vi "Launch New Client Proxy.vi"(8 "error in (no error)":errorcluster, 9 "Client Proxy LNA":refnum<class "Client Proxy LNA.lvclass">, 10 "remote address":string, 11 "Server Controller in":refnum<class "Server Controller.lvclass">) -> (0 "error out":errorcluster, 3 "Server Controller out":refnum<class "Server Controller.lvclass">)   [LabVIEW 2016]
uses:
  Server Controller.lvclass
  Client Proxy LNA/Client Proxy LNA.lvclass
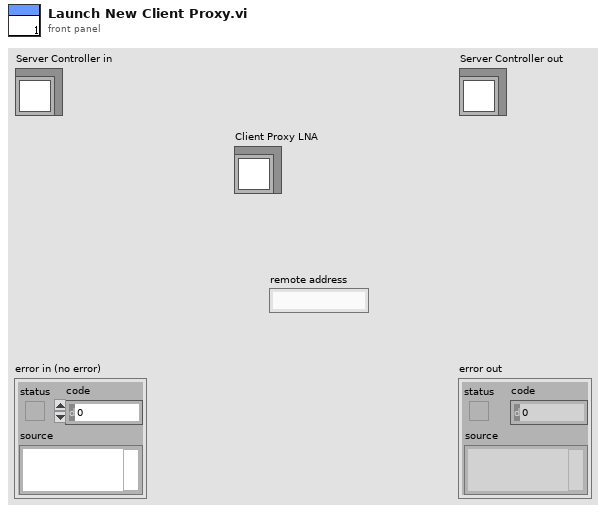
[diagram p1: front panel]
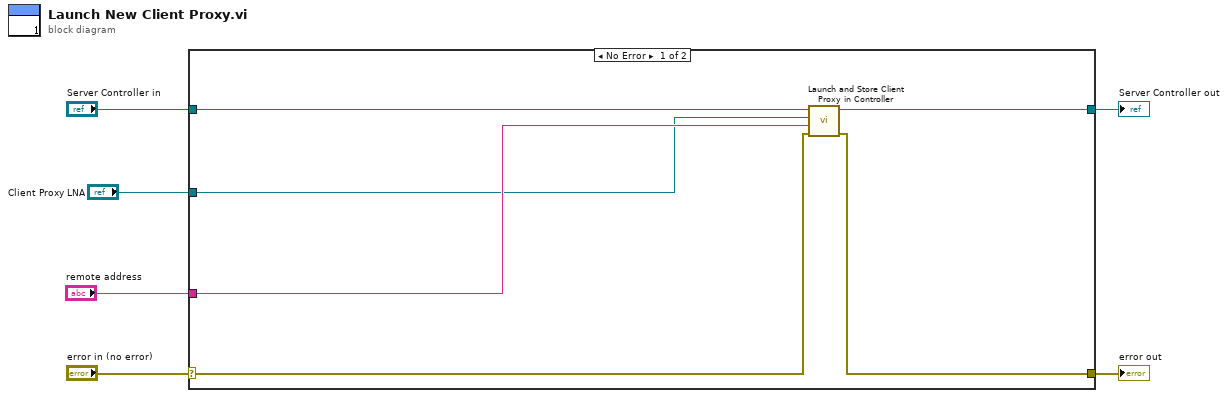
[diagram p0: block diagram]
diagram:
  n1 = case shown="No Error" "error in (no error)" {
    selector: "error in (no error)" -> [w12 w14]
    tunnel: [w11 w14] -> w5
    tunnel: [w9 w13] -> w3
    tunnel: "Server Controller in" -> [w10 w13]
    tunnel: "remote address" -> [w8 _]
    tunnel: "Client Proxy LNA" -> [w7 _]
    frame No Error {
      n2 = call "Launch and Store Client Proxy in Controller.vi"("error in (no error)"=w12, 9:w8, "Network Actor in"=w7, "Server Controller in"=w10) -> ("error out"=w11:errorcluster, "Server Controller Out"=w9:refnum<class "Server Controller.lvclass">)  [unwired: 6 in]
    }
    frame Error {
    }
  }
  "error out" <- w5
  "Server Controller out" <- w3
